vi "ErrorCombiner.vi"(8 "Return In":i32, 11 "error in (no error)":errorcluster) -> (0 "Return Out":i32, 3 "error out":errorcluster)   [LabVIEW 2011]
panel:
  # "ERROR Combiner"
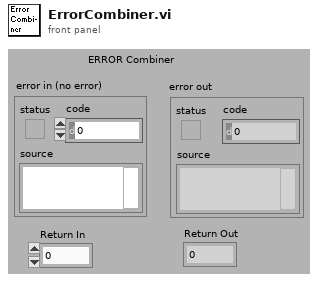
[diagram p1: front panel]
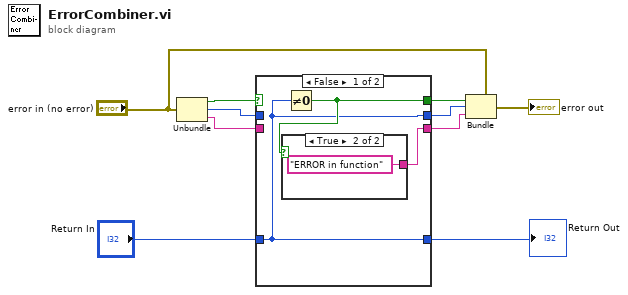
[diagram p0: block diagram]
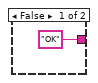
[diagram p2: hidden frame]
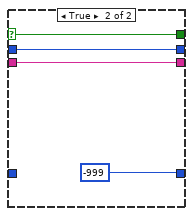
[diagram p3: hidden frame]
diagram:
  n1 = Unbundle("error in (no error)") -> ("status"=w8:bool, "code"=w6:i32, "source"=w5:string)
  n2 = case shown="False" w8 {
    selector: w8 -> [_ w19]
    tunnel: [w11 w18] -> w7
    tunnel: w6 -> [_ w18]
    tunnel: w5 -> [_ w17]
    tunnel: [w13 w17] -> w4
    tunnel: [w12 w19] -> w3
    tunnel: "Return In" -> [w11 _]
    tunnel: [w11 i16 -999 ("Return In")] -> w1
    frame False {
      n3 = Not Equal To 0?(x=w11) -> (x != 0?=w12:bool)
      n4 = case shown="True" w12 {
        tunnel: ["OK" ("source") "ERROR in function" ("source")] -> w13
        frame False {
        }
        frame True {
        }
      }
    }
    frame True {
    }
  }
  "Return Out" <- w1
  n5 = Bundle(cluster="error in (no error)", "status"=w3, "code"=w7, "source"=w4) -> (→"error out":errorcluster)
